vi "MesaurementModus.vi"() -> ()   [LabVIEW 2013]
panel:
  in  "ModusMesaurement":enum32{"Fast", "Step"}(radio)
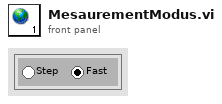
[diagram p1: front panel]
diagram:
